vi "ExtractTimeout.vi"(0 "Input Params":string[](array[string]), 3 "Default Timeout":i32=5000) -> (7 "Timeout":i32, 10 "Remaining Params":string[](array[string]))   [LabVIEW 2018, in "Test.lvclass"]
uses:
  Test.lvclass
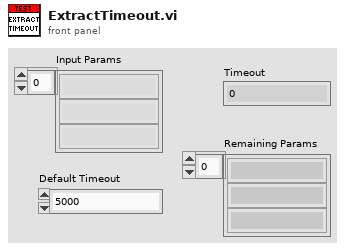
[diagram p1: front panel]
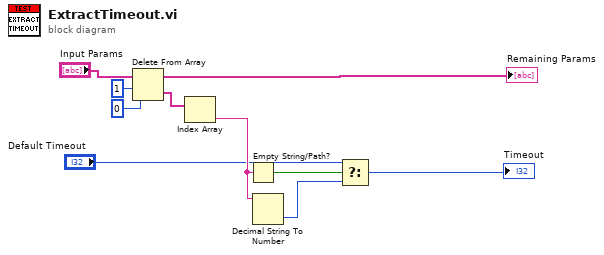
[diagram p0: block diagram]
diagram:
  n1 = Delete From Array(array="Input Params", length=1, index=0) -> (deleted portion=w6:string[], array with subset deleted=→"Remaining Params":string[])
  n2 = Index Array(array=w6) -> (element=w5:string)  [unwired: 1 in]
  n3 = Empty String/Path?(string/path=w5) -> (empty?=w4:bool)
  n4 = Decimal String To Number(string=w5) -> (number=w3:i32)  [unwired: 2 in, 1 out]
  n5 = Select(t="Default Timeout", s=w4, f=w3) -> (s? t:f=→"Timeout":i32)
